vi "getWidth.vi"(0 "HGF_IMAQDevice in":refnum<class "HGF_IMAQDevice.lvclass">, 5 "error in (no error)":errorcluster) -> (14 "HGF_IMAQDevice out":refnum<class "HGF_IMAQDevice.lvclass">, 17 "Width":i32, 19 "error out":errorcluster)   [LabVIEW 2014, in "HGF_IMAQ.lvlib" / "HGF_IMAQDevice.lvclass"]
doc: "Returns the width of the image taken by the camera."
uses:
  HGF_IMAQDevice.lvclass
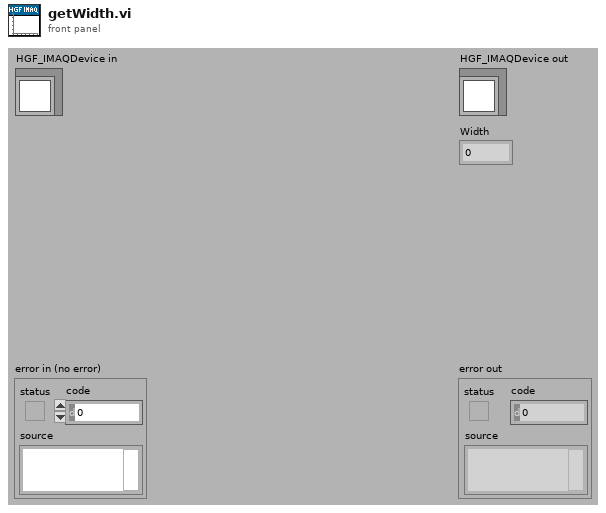
[diagram p1: front panel]
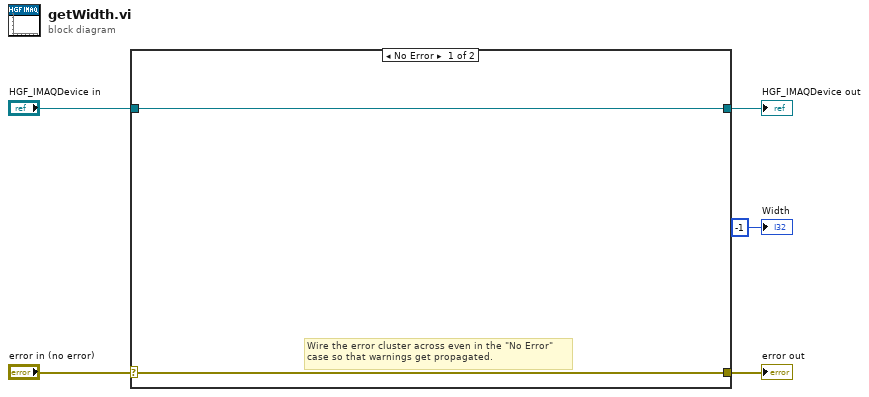
[diagram p0: block diagram]
diagram:
  n1 = case shown="No Error" "error in (no error)" {
    selector: "error in (no error)" -> [w6 w9]
    tunnel: [w6 w9] -> w4
    tunnel: [w7 w8] -> w2
    tunnel: "HGF_IMAQDevice in" -> [w7 w8]
    frame No Error {
      # "Wire the error cluster across even in the \"No Error\"\ncase so that warnings get propagated."
    }
    frame Error {
    }
  }
  "error out" <- w4
  "HGF_IMAQDevice out" <- w2
  "Width" <- -1 ("Width")
